vi "array.vi"() -> ()   [LabVIEW 2018]
panel:
  in  "stop":bool
  in  "Array":string[](array[string])
  out "Array_Copy":string[](array[string])
  out "Sorted Array":string[](array[string])
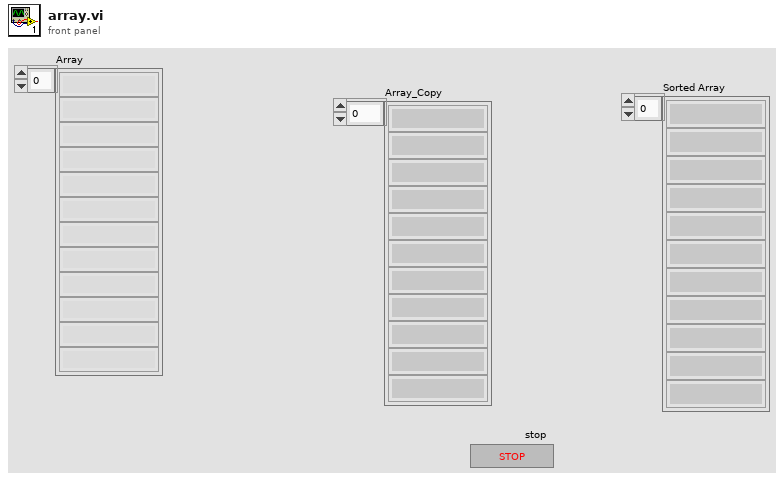
[diagram p1: front panel]
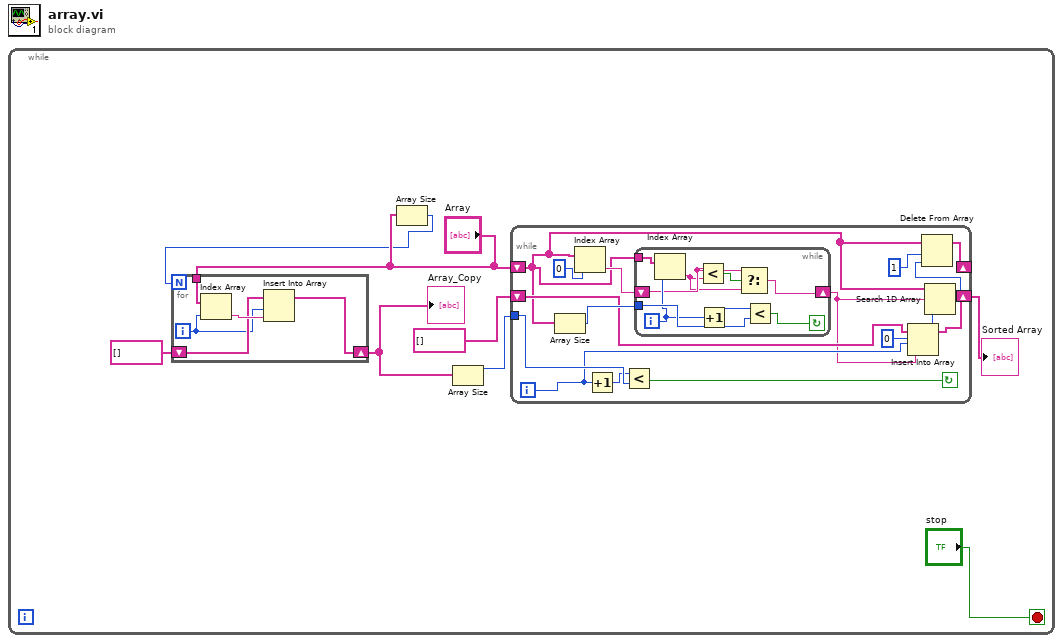
[diagram p0: block diagram]
diagram:
  n1 = while {
    stop <- "stop" stop-if-true
    n2 = Array Size(array="Array") -> (size(s)=w3:i32)
    n3 = for {
      N: w3 -> [_]
      tunnel: "Array" -> [w13]
      shift-right: [w10] -> w6
      shift-left: string[] [] -> [w11]
      i -> [w9]
      n4 = Index Array(array=w13, index=w9) -> (element=w12:string)
      n5 = Insert Into Array(array=w11, index=w9, new element=w12) -> (w10:string[])
    }
    "Array_Copy" <- w6
    n6 = Array Size(array=w6) -> (size(s)=w2:i32)
    n7 = while {
      shift-right: [w18] -> _
      shift-left: "Array" -> [w14]
      shift-right: [w15] -> w5
      shift-left: string[] [] -> [w21]
      tunnel: w2 -> [w27]
      i -> [w22]
      stop <- w28 continue-if-true
      n8 = Array Size(array=w14) -> (size(s)=w26:i32)
      n9 = Index Array(array=w14, index=0) -> (element=w24:string)
      n10 = Increment(x=w22) -> (x+1=w25:i32)
      n11 = Less?(x=w25, y=w27) -> (x < y?=w28:bool)
      n12 = while {
        tunnel: w14 -> [w37]
        tunnel: w26 -> [w35]
        shift-right: [w31] -> w17
        shift-left: w24 -> [w30]
        i -> [w32]
        stop <- w36 continue-if-true
        n13 = Index Array(array=w37, index=w32) -> (element=w29:string)
        n14 = Less?(x=w30, y=w29) -> (x < y?=w33:bool)
        n15 = Increment(x=w32) -> (x+1=w34:i32)
        n16 = Select(t=w30, s=w33, f=w29) -> (s? t:f=w31:string)
        n17 = Less?(x=w34, y=w35) -> (x < y?=w36:bool)
      }
      n18 = Insert Into Array(array=w21, index=w22, new element=w17) -> (w15:string[])
      n19 = Search 1D Array(1D array=w14, element=w17, start index (0)=0) -> (index of element=w19:i32)
      n20 = Delete From Array(array=w14, length=1, index=w19) -> (array with subset deleted=w18:string[])  [unwired: 1 out]
    }
    "Sorted Array" <- w5
  }
